vi "Get Visible (Label).vi"(8 "error in (no error)":errorcluster, 10 "Label":string, 11 "Interaction By Refererence in":refnum<class "Interaction By Refererence.lvclass">) -> (0 "error out":errorcluster, 1 "Match?":bool, 2 "Visible?":bool, 3 "Interaction By Refererence out":refnum<class "Interaction By Refererence.lvclass">, 4 "Item visible?":bool)   [LabVIEW 2021, in "Interaction By Refererence.lvclass"]
uses:
  Interaction By Refererence.lvclass
  Interaction By Refererence.lvclass/Interaction By Refererence.ctl
  IContainer/Interaction/Interaction.lvclass
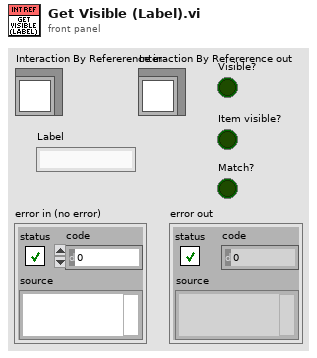
[diagram p1: front panel]
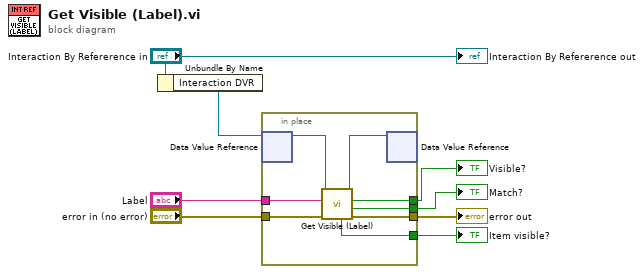
[diagram p0: block diagram]
diagram:
  n1 = Unbundle By Name("Interaction By Refererence in") -> ("Interaction DVR"=w1:refnum<data-value>)
  n2 = in-place {
    in-place-border: [w16] -> w8
    in-place-border: [w15] -> w7
    in-place-border: [w14] -> w6
    in-place-border: [w13] -> w5
    in-place-border: "error in (no error)" -> [w12]
    in-place-border: "Label" -> [w11]
    n3 = in-place-dvr #1(w1) -> (w10:refnum<class "Interaction.lvclass">)  [unwired: 1 out]
    n4 = call-dynamic "Get Visible (Label).vi"("error in (no error)"=w12, "Label"=w11, "IContainer in"=w10) -> ("error out"=w16:errorcluster, "Match?"=w15:bool, "Visible?"=w14:bool, "IContainer out"=w9:refnum<class "Interaction.lvclass">, "Item visible?"=w13:bool)  [unwired: 4 in]
    n5 = in-place-dvr #1(w9) -> ()  [unwired: 2 out]
  }
  "error out" <- w8
  "Visible?" <- w6
  "Item visible?" <- w5
  "Match?" <- w7
  "Interaction By Refererence out" <- "Interaction By Refererence in"
